vi "VI Ref Or Path.vi"(8 "Error In":errorcluster, 10 "VI Path":path, 11 "VI Ref":refnum<vi>) -> (0 "Error Out":errorcluster, 3 "VI out":refnum<vi>)   [LabVIEW 2020, in "LMH-Toolbox.lvlib" / "LMH-Front-Panel-Clean-Up.lvlib"]
doc: "Returns the VI Ref if wired or\nA VI Ref to the VI in the VI Path control or\nReturns an error if neither of the above are valid."
uses:
  LMH-Front-Panel-Clean-Up.lvlib
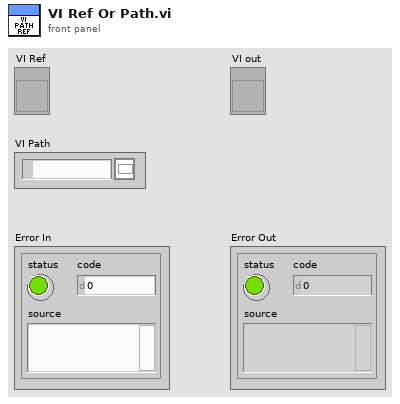
[diagram p1: front panel]
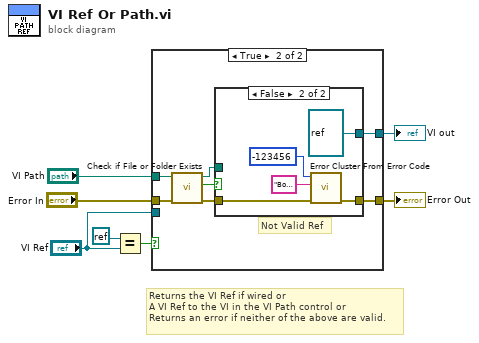
[diagram p0: block diagram]
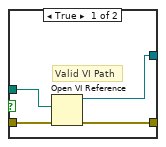
[diagram p3: hidden frame]
diagram:
  # "Returns the VI Ref if wired or\nA VI Ref to the VI in the VI Path control or\nReturns an error if neither of the above are valid."
  n1 = Equal?(x=refnum<k0> refnum, y="VI Ref") -> (x = y?=w2:bool)
  n2 = case shown="True" w2 {
    tunnel: "VI Path" -> [_ w16]
    tunnel: "Error In" -> [w8 w15]
    tunnel: [w8 w11] -> w6
    tunnel: [w9 w10] -> w5
    tunnel: "VI Ref" -> [w9 _]
    frame False {
      # "Valid VI Ref"
    }
    frame True {
      # "Not Valid Ref"
      n3 = call <vilib>:"Check if File or Folder Exists.vi"("error in (no error)"=w15, "path"=w16) -> ("error out"=w14:errorcluster, "file or folder exists?"=w12:bool, "dup path"=w13:path)  [unwired: 7 in]
      n4 = case shown="False" w12 {
        tunnel: w14 -> [w19 w24]
        tunnel: w13 -> [w20 _]
        tunnel: [w18 w23] -> w11
        tunnel: [w17 refnum<vi> refnum ("vi reference")] -> w10
        frame True {
          # "Valid VI Path"
          n5 = Open VI Reference(vi path=w20, error in (no error)=w19) -> (vi reference=w17:refnum<vi>, error out=w18:errorcluster)  [unwired: 4 in]
        }
        frame False {
          n6 = call <vilib>:"Error Cluster From Error Code.vi"("error in (no error)"=w24, "error message (\"\")"="Both VI Path and VI Ref are invalid." ("error message (\"\")"), "error code (0)"=-123456) -> ("error out"=w23:errorcluster)  [unwired: 6 in]
        }
      }
    }
  }
  "Error Out" <- w6
  "VI out" <- w5
